vi "CANShark_DeviceClose.vi"(11 "Device Handler":i64) -> (3 "Device close value":i32)   [LabVIEW 2026]
uses:
  x64/Release/CanSharkApi_Dll1.dll
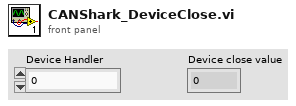
[diagram p1: front panel]
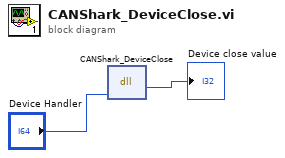
[diagram p0: block diagram]
diagram:
  n1 = dll-call lib="C:/Users/TECQNIO/Documents/CANSHARK LABVIEW API PACKAGE/x64/Release/CanSharkApi_Dll1.dll" fn="CANShark_DeviceClose"("Device"="Device Handler") -> ("return type"=→"Device close value":i32)  [unwired: 4 in, 2 out]
